vi "PXI-Update AO.vi"(0 "AO Tasks":T2[](array[typedef]), 5 "Wait for Buffer Space (T)?":bool=TRUE, 7 "AO Waveforms":dbl[][](array[numeric]), 11 "error in (no error)":errorcluster, 12 "DAQ Write State":T1) -> (8 "PauseDAQ":bool, 14 "DAQ Write State Out":T1, 15 "error out":errorcluster)   [LabVIEW 2020]
uses:
  Type Defs/Task Struct.ctl
  Type Defs/DAQ Write State enum.ctl
  PXI Globals.vi
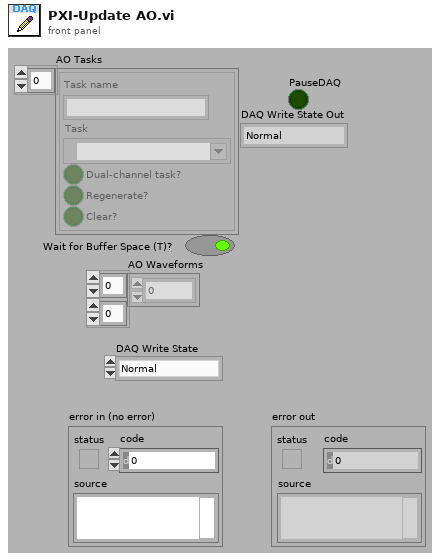
[diagram p1: front panel]
types:
  T1 = typedef "DAQ Write State enum.ctl" = enum16{"Normal", "Ramp down", "Zero buffers", "Done"}
  T2 = typedef "Task Struct.ctl" = cluster{"Task name":string, "Task":refnum<k21>, "Dual-channel task?":bool, "Regenerate?":bool, "Clear?":bool}
  T3 = typedef "Ramping Params.ctl" = cluster{"Ramp up?":bool, "Ramp down?":bool, "Ramp duration (msecs)":dbl, "Ramp type":enum16{"Linear", "Cos2"}}
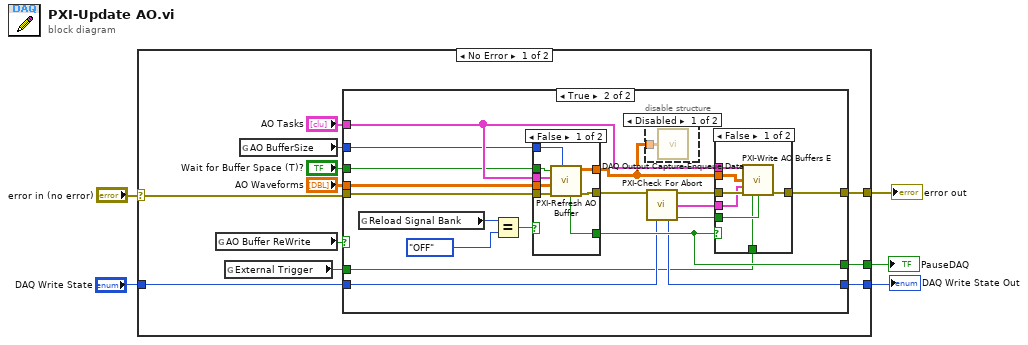
[diagram p0: block diagram]
diagram:
  n1 = case shown="No Error" "error in (no error)" {
    selector: "error in (no error)" -> [w13 w57]
    tunnel: [w16 w57] -> w5
    tunnel: [w10 _] -> w3
    tunnel: "DAQ Write State" -> [w8 w56]
    tunnel: [w7 w56] -> w1
    frame No Error {
      n2 = global read "PXI Globals.vi" "AO Buffer ReWrite"() -> (w11:bool)
      n3 = global read "PXI Globals.vi" "External Trigger"() -> (w6:bool)
      n4 = global read "PXI Globals.vi" "AO BufferSize"() -> (w12:i32)
      n5 = case shown="True" w11 {
        tunnel: "AO Tasks" -> [_ w34]
        tunnel: w13 -> [w18 w33]
        tunnel: [w18 w35] -> w16
        tunnel: "AO Waveforms" -> [_ w36]
        tunnel: w12 -> [_ w30]
        tunnel: [_ w28] -> w10
        tunnel: "Wait for Buffer Space (T)?" -> [_ w27]
        tunnel: w8 -> [w17 w24]
        tunnel: [w17 w21] -> w7
        tunnel: w6 -> [_ w19]
        frame False {
        }
        frame True {
          n6 = global read "PXI Globals.vi" "Reload Signal Bank"() -> (w31:enum32{"OFF", "ENABLED", "FORCED"})
          n7 = Equal?(x=w31, y=enum16{"OFF", "ENABLED", "FORCED"}."OFF") -> (x = y?=w29:bool)
          n8 = case shown="False" w29 {
            tunnel: w33 -> [w53 w55]
            tunnel: w36 -> [w52 w54]
            tunnel: [w51 w54] -> w20
            tunnel: [w50 w55] -> w26
            tunnel: w34 -> [w49 _]
            tunnel: w30 -> [w48 _]
            tunnel: [w47 _] -> w28
            tunnel: w27 -> [w46 _]
            frame False {
              n9 = call "PXI-Refresh AO Buffer.vi"("BufferSize"=w48, "error in (no error)"=w53, "AO Waveforms In"=w52, "AO Tasks"=w49, "Wait for buffer space? (T)"=w46) -> ("error out (no error)"=w50:errorcluster, "AO Waveforms Out"=w51:dbl[][], "PauseDAQ"=w47:bool)  [unwired: 4 in]
            }
            frame True {
            }
          }
          n10 = disable-structure shown="Disabled" {
            disable-tunnel: w20 -> [w37 _]
            frame Disabled {
              n11 = call "DAQ Output Capture-Enqueue Data.vi"("Data"=w37) -> ()  [unwired: 14 in, 1 out]
            }
            frame Enabled {
            }
          }
          n12 = call "PXI-Check For Abort.vi"("error in (no error)"=w26, "DAQ Write State"=w24) -> ("error out"=w25:errorcluster, "Ramping"=w23:T3, "DAQ Write State Out"=w21:T1, "Zero?"=w22:bool)  [unwired: 10 in]
          n13 = case shown="False" w28 {
            tunnel: [w44 w45] -> w35
            tunnel: w20 -> [w43 _]
            tunnel: w25 -> [w42 w45]
            tunnel: w34 -> [w41 _]
            tunnel: w23 -> [w40 _]
            tunnel: w22 -> [w39 _]
            tunnel: w19 -> [w38 _]
            frame False {
              n14 = call "PXI-Write AO Buffers E.vi"("AO Tasks"=w41, "AO Waveforms"=w43, "Ramping"=w40, "error in (no error)"=w42, "Force write"=w38, "zero output"=w39) -> ("error out"=w44:errorcluster)  [unwired: 8 in, 1 out]
            }
            frame True {
            }
          }
        }
      }
    }
    frame Error {
    }
  }
  "error out" <- w5
  "PauseDAQ" <- w3
  "DAQ Write State Out" <- w1
